vi "Menu Click.vi"(8 "error in (no error)":errorcluster, 10 "MenuData":T1, 11 "CallActorCenter in":refnum<class "CallActorCenter.lvclass">) -> (0 "error out":errorcluster, 3 "CallActorCenter out":refnum<class "CallActorCenter.lvclass">)   [LabVIEW 2021]
uses:
  CallActorCenter.lvclass
  C:/Program Files (x86)/National Instruments/LabVIEW 2021/user.lib/John_Lib/AbstractActorTemplate/AbstractActorTemplate/UIActorTop.lvclass
  Source_Public/Public Interface/MenuProcess/MenuData.ctl
  Source_Public/Public Interface/InsertRightSubPanel Messages/Insert Right SubPanel Msg/Insert Right SubPanel Msg.lvclass/Insert Right SubPanel Msg.ctl
  <vilib>/ActorFramework/Message Enqueuer/Message Enqueuer.lvclass/Message Enqueuer.ctl
  <vilib>/ActorFramework/Message Enqueuer/Enqueue.vi
  Source_Public/Public Interface/InsertRightSubPanel Messages/Insert Right SubPanel Msg/Insert Right SubPanel Msg.lvclass
  C:/Program Files (x86)/National Instruments/LabVIEW 2021/vi.lib/ActorFramework/Message/Message.lvclass
  Interface/SaveSequence Messages/Save Sequence Msg/Save Sequence Msg.lvclass
  <vilib>/ActorFramework/Message Priority Queue/Priority Enqueue.vi
  <vilib>/ActorFramework/Message Enqueuer/Message Enqueuer.lvclass
  Source_Public/Public Interface/MenuProcess/MenuProcess.lvclass
panel:
  out "MenuData 2":T1
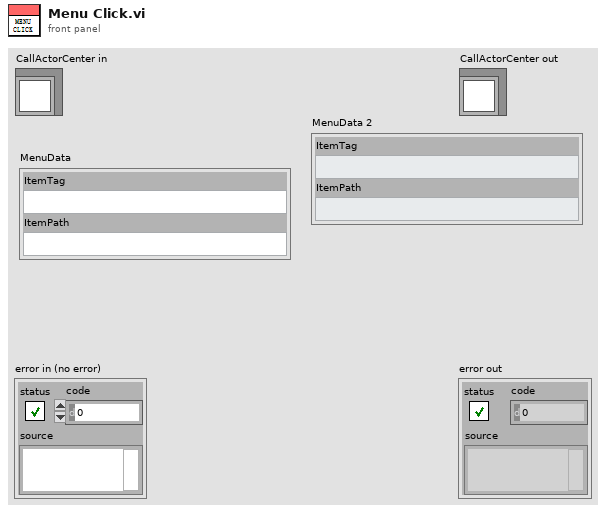
[diagram p1: front panel]
types:
  T1 = typedef "MenuProcess.lvclass/MenuData.ctl" = cluster{"ItemTag":string, "ItemPath":string}
  T2 = map{string, refnum<class "Message Enqueuer.lvclass">}
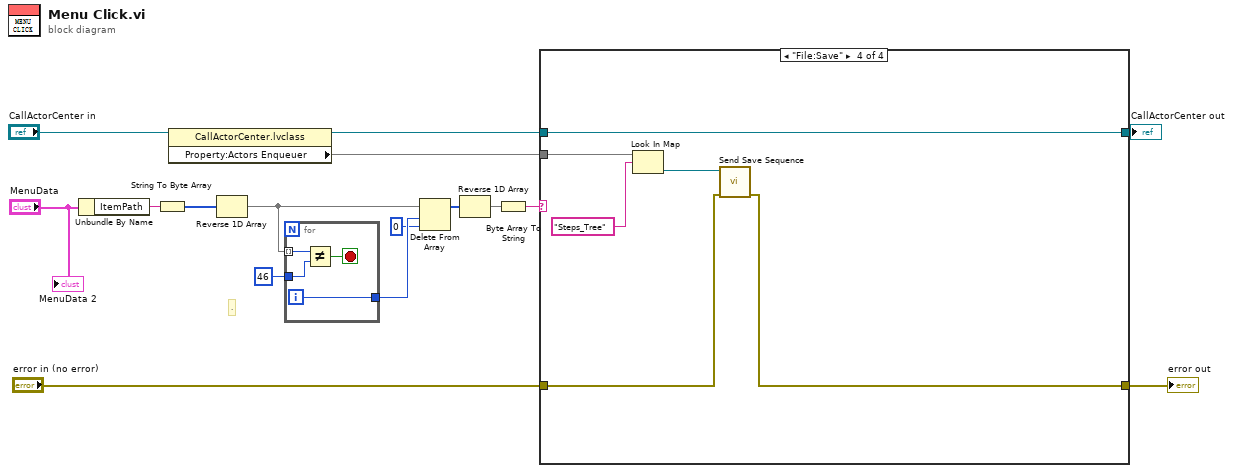
[diagram p0: block diagram]
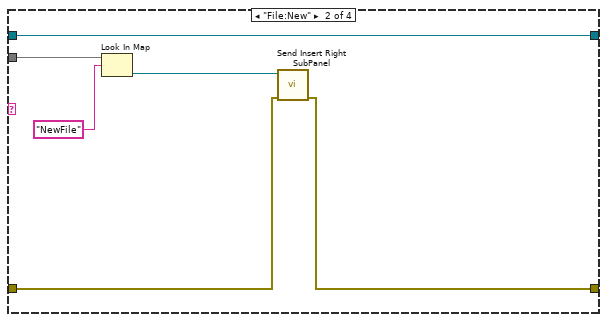
[diagram p3: hidden frame]
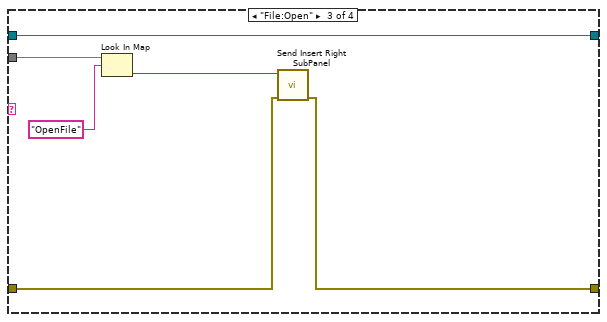
[diagram p4: hidden frame]
diagram:
  # "."
  n1 = Unbundle By Name("MenuData") -> ("ItemPath"=w6:string)
  n2 = String To Byte Array(string=w6) -> (unsigned byte array=w13:u8[])
  n3 = property class="CallActorCenter.lvclass"(reference="CallActorCenter in") -> (reference out=w3:refnum<class "CallActorCenter.lvclass">, "Property:Actors Enqueuer"=w2:T2)  [unwired: 1 in, 1 out]
  n4 = Reverse 1D Array(array=w13) -> (reversed array=w11:u8[])
  n5 = for {
    tunnel: w11 -> [w20] mode=indexing
    tunnel: u8 46 ("y") -> [w19]
    tunnel: [w18] -> w10
    i -> [w18]
    stop <- w17 stop-if-true
    n6 = Not Equal?(x=w20, y=w19) -> (x != y?=w17:bool)
  }
  n7 = Delete From Array(array=w11, length=w10, index=0) -> (array with subset deleted=w8:u8[])  [unwired: 1 out]
  n8 = Reverse 1D Array(array=w8) -> (reversed array=w7:u8[])
  n9 = Byte Array To String(unsigned byte array=w7) -> (string=w5:string)
  n10 = case shown="\"File:Save\"" w5 {
    tunnel: w3 -> [w22 w28 w34 w40]
    tunnel: [w22 w28 w34 w40] -> w14
    tunnel: "error in (no error)" -> [w21 w24 w30 w36]
    tunnel: w2 -> [_ w27 w33 w39]
    tunnel: [w21 w23 w29 w35] -> w1
    frame "False", Default {
    }
    frame "File:New" {
      n11 = Look In Map(map=w27, key="NewFile") -> (value=w25:refnum<class "Message Enqueuer.lvclass">)  [unwired: 1 in, 1 out]
      n12 = call "Send Insert Right SubPanel.vi"("error in (no error)"=w24, "Message Enqueuer"=w25) -> ("error out"=w23:errorcluster)  [unwired: 8 in, 1 out]
    }
    frame "File:Open" {
      n13 = Look In Map(map=w33, key="OpenFile") -> (value=w31:refnum<class "Message Enqueuer.lvclass">)  [unwired: 1 in, 1 out]
      n14 = call "Send Insert Right SubPanel.vi"("error in (no error)"=w30, "Message Enqueuer"=w31) -> ("error out"=w29:errorcluster)  [unwired: 8 in, 1 out]
    }
    frame "File:Save" {
      n15 = Look In Map(map=w39, key="Steps_Tree") -> (value=w37:refnum<class "Message Enqueuer.lvclass">)  [unwired: 1 in, 1 out]
      n16 = call "Send Save Sequence.vi"("error in (no error)"=w36, "Message Enqueuer"=w37) -> ("error out"=w35:errorcluster)  [unwired: 8 in, 1 out]
    }
  }
  "error out" <- w1
  "CallActorCenter out" <- w14
  "MenuData 2" <- "MenuData"
